vi "LV String to utf8 String.vi"(8 "错误输入":errorcluster, 11 "Input String":string) -> (0 "错误输出":errorcluster, 3 "Output String":string)   [LabVIEW 2012, in "Encoding.lvlib"]
uses:
  Encoding.lvlib
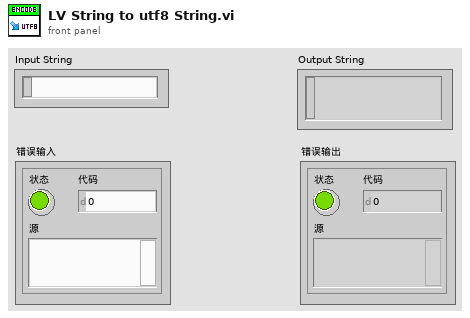
[diagram p1: front panel]
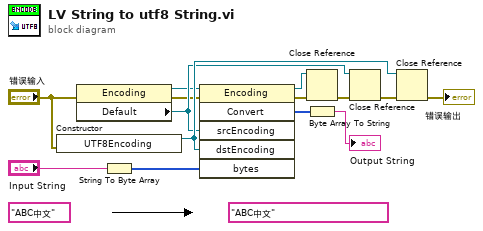
[diagram p0: block diagram]
diagram:
  (unwired) "ABC中文" ("Output String")
  (unwired) "ABC中文" ("Input String")
  n1 = constructor class="UTF8Encoding"(error in="错误输入") -> (reference out=w14:refnum<k24>)  [unwired: 2 in, 2 out]
  n2 = property class="Encoding"(error in="错误输入") -> (reference out=w9:refnum<k24>, error out=w8:errorcluster, "Default"=w10:refnum<k24>)  [unwired: 1 in]
  n3 = String To Byte Array(string="Input String") -> (unsigned byte array=w6:u8[])
  n4 = invoke class="Encoding" method="Convert"(reference=w9, error in=w8, "srcEncoding"=w10, "dstEncoding"=w14, "bytes"=w6) -> (reference out=w1:refnum<k24>, error out=w2:errorcluster, "Convert"=w3:u8[])  [unwired: 1 in, 3 out]
  n5 = Close Reference(reference=w1, error in (no error)=w2) -> (error out=w11:errorcluster)
  n6 = Byte Array To String(unsigned byte array=w3) -> (string=→"Output String":string)
  n7 = Close Reference(reference=w10, error in (no error)=w11) -> (error out=w12:errorcluster)
  n8 = Close Reference(reference=w14, error in (no error)=w12) -> (error out=→"错误输出":errorcluster)
